vi "niccc-labview-xygraph.vi"() -> ()   [LabVIEW 2020]
uses:
  Controls/Frame Info (XY Graph).ctl
  Controls/Vertex.ctl
  Controls/State.ctl
panel:
  in  "FPS":u32=20
  in  "Slow Draw":bool
  out "Frame":i32
  out "XY Graph":cluster{"x":dbl[], "y":dbl[]}[](graph)
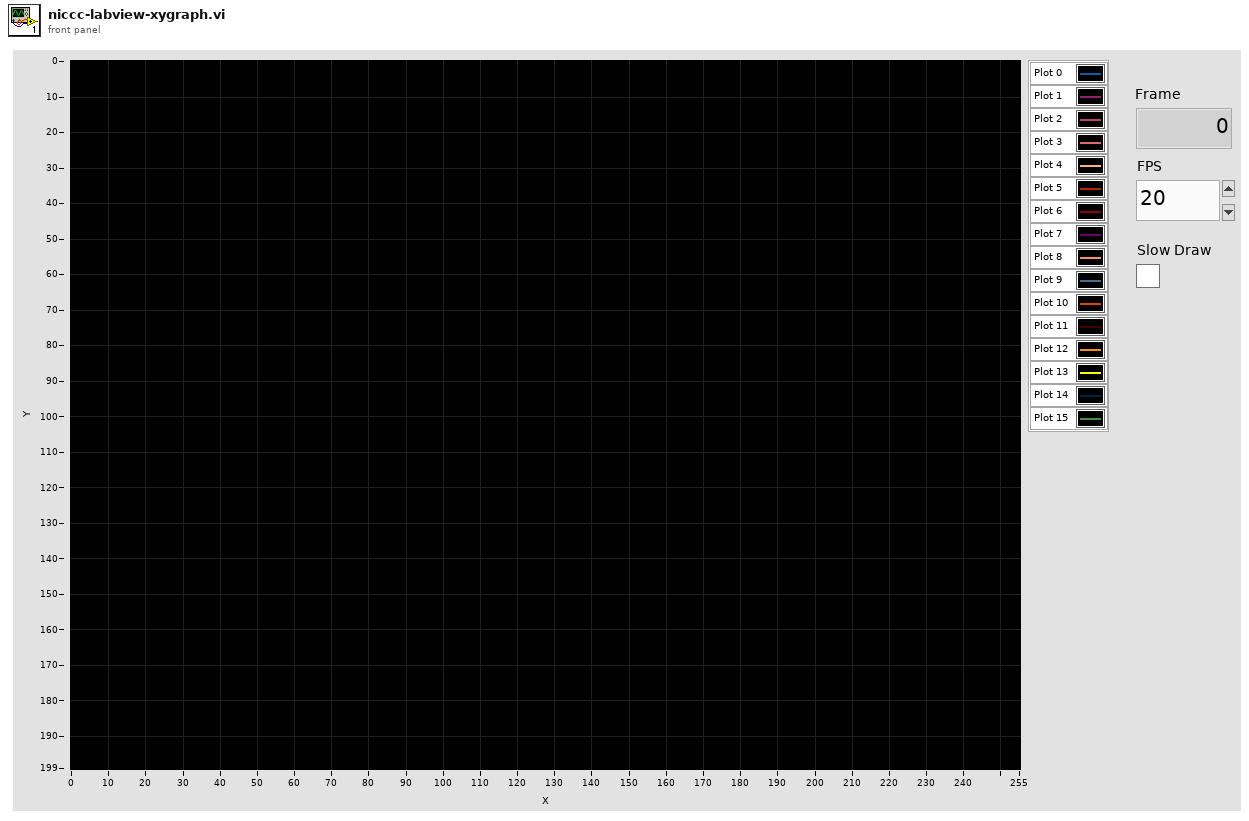
[diagram p1: front panel]
types:
  T1 = typedef "Frame Info (XY Graph).ctl" = cluster{"Clear Screen":bool, "Palette Data":bool, "Indexed":bool, "Indexed Verts":T2[], "Frame":i32, "Plots":cluster{"x":dbl[], "y":dbl[]}[]}
  T2 = typedef "Vertex.ctl" = cluster{"x":u8, "y":u8}
  T3 = typedef "State.ctl" = enum16{"Init", "Read Flags", "Clear Screen", "Update Palette", "Read Indexed", "Draw Polygons", "Skip 64kB", "Finish"}
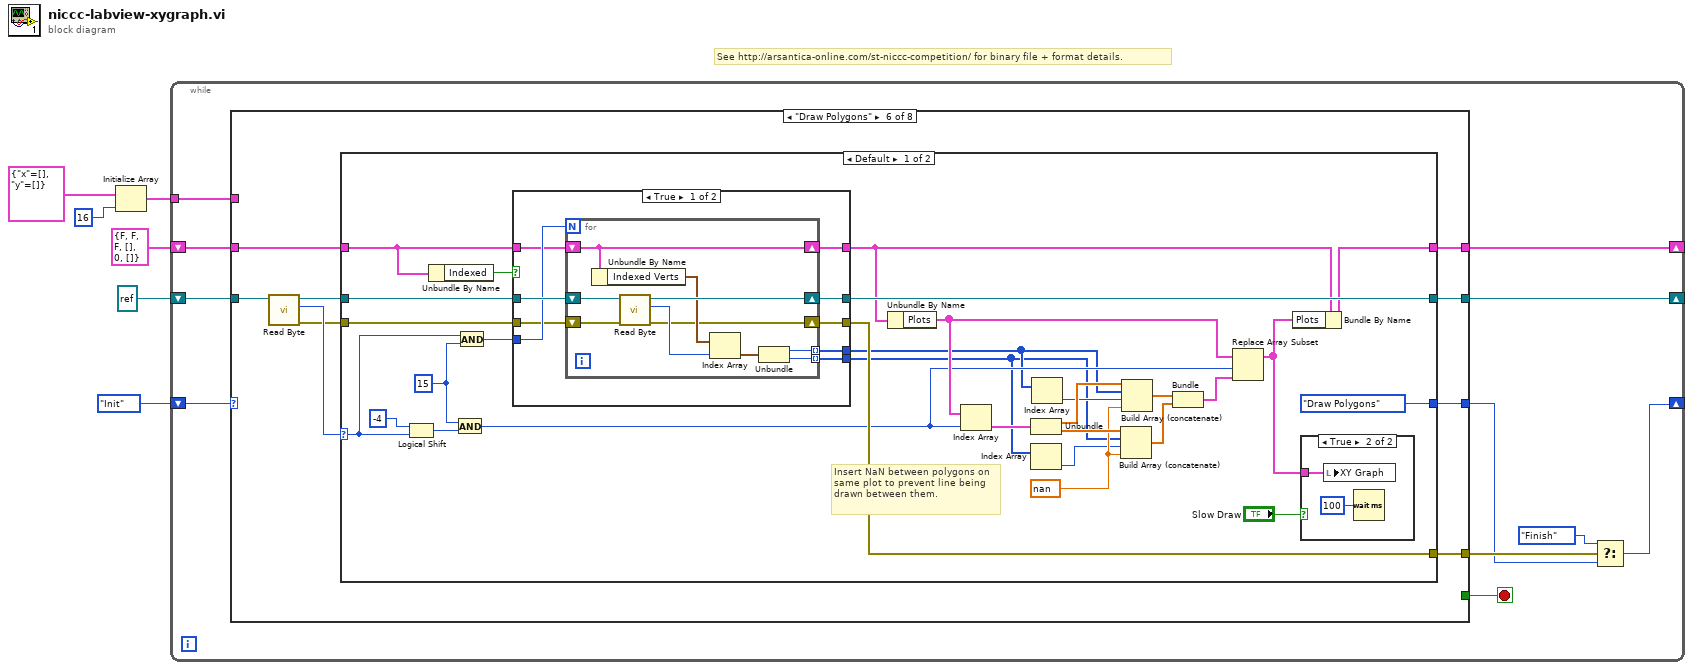
[diagram p0: block diagram]
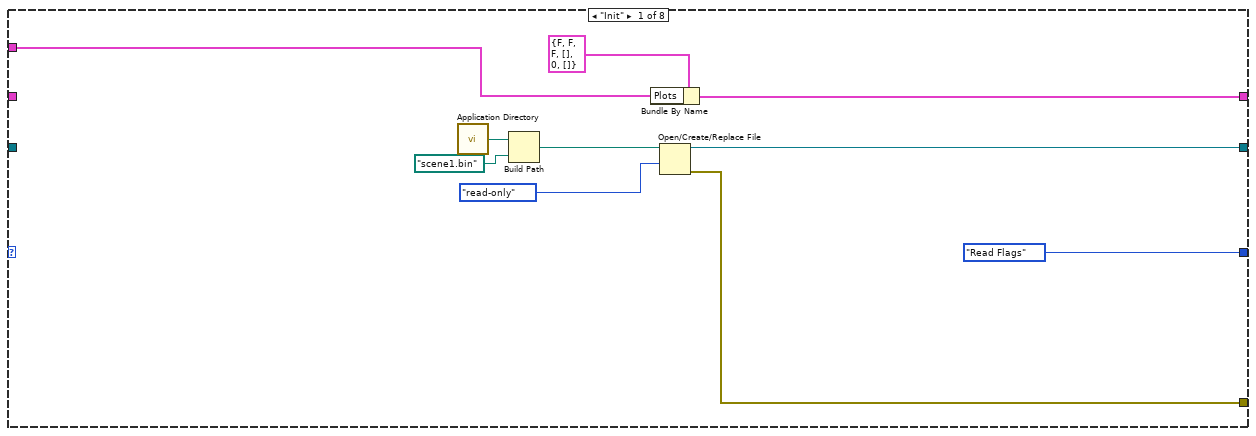
[diagram p2: hidden frame]
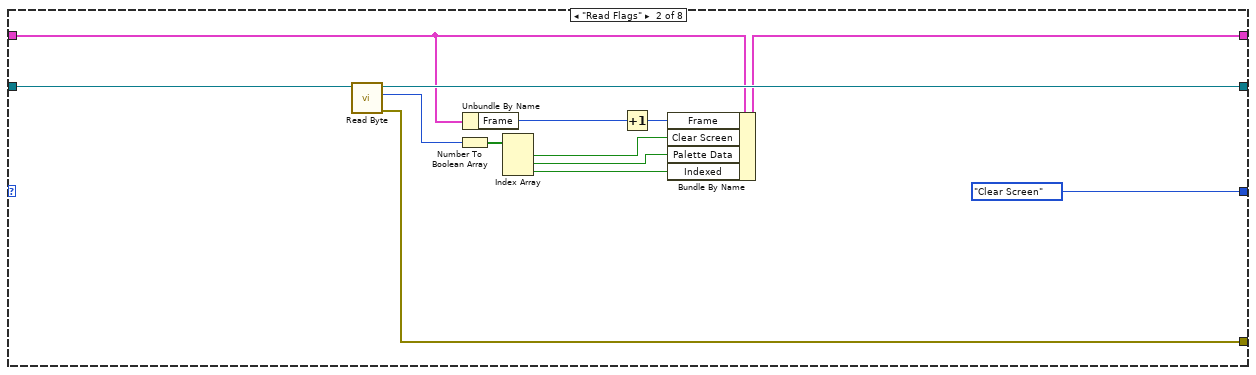
[diagram p3: hidden frame]
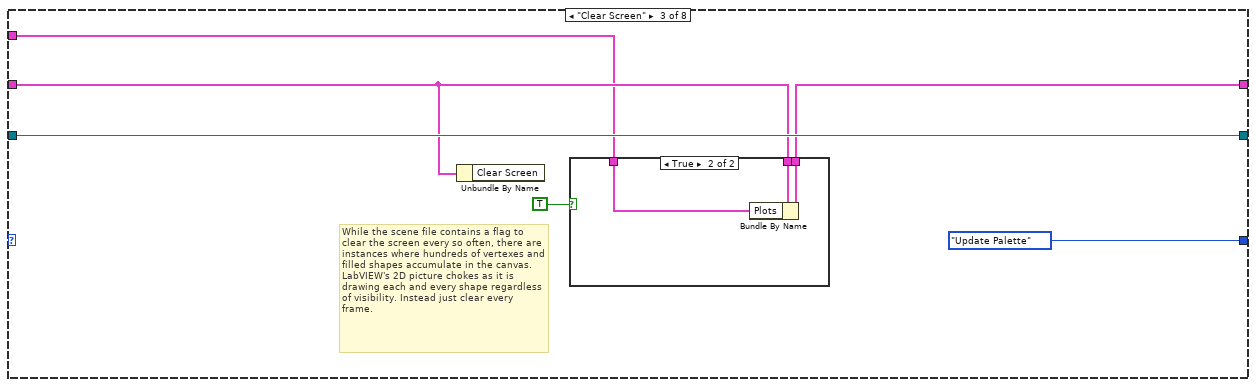
[diagram p4: hidden frame]
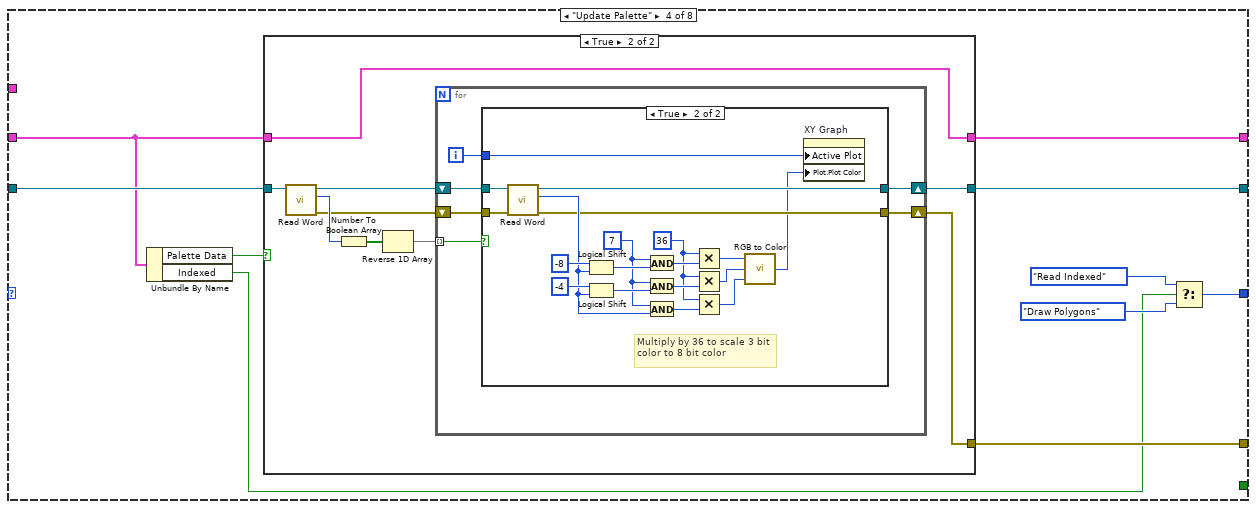
[diagram p6: hidden frame]
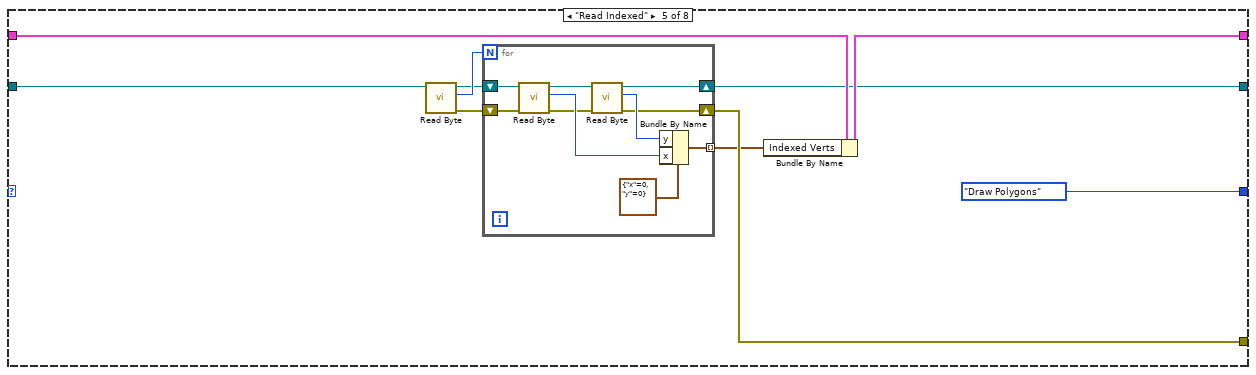
[diagram p9: hidden frame]
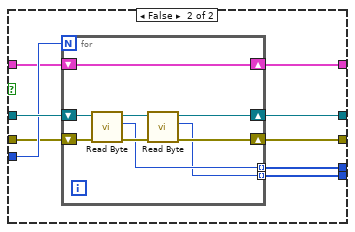
[diagram p11: hidden frame]
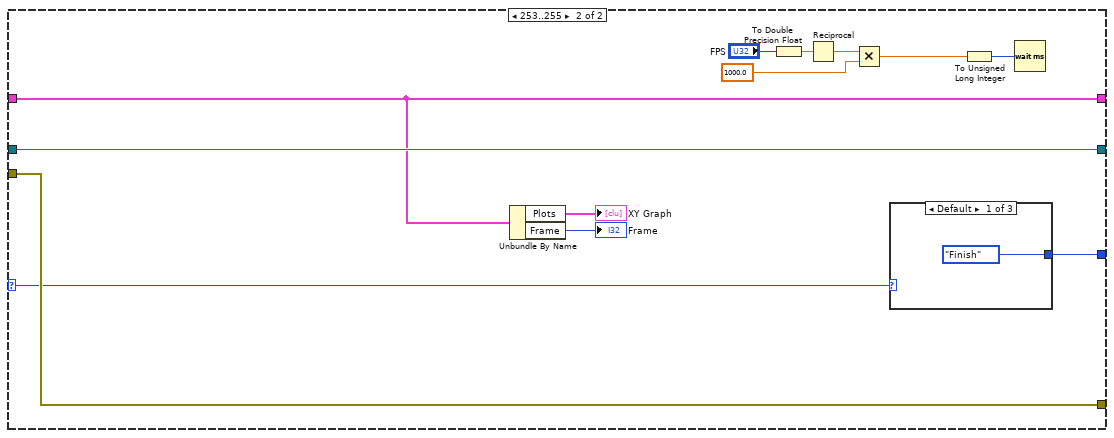
[diagram p12: hidden frame]
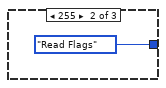
[diagram p13: hidden frame]
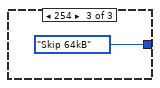
[diagram p14: hidden frame]
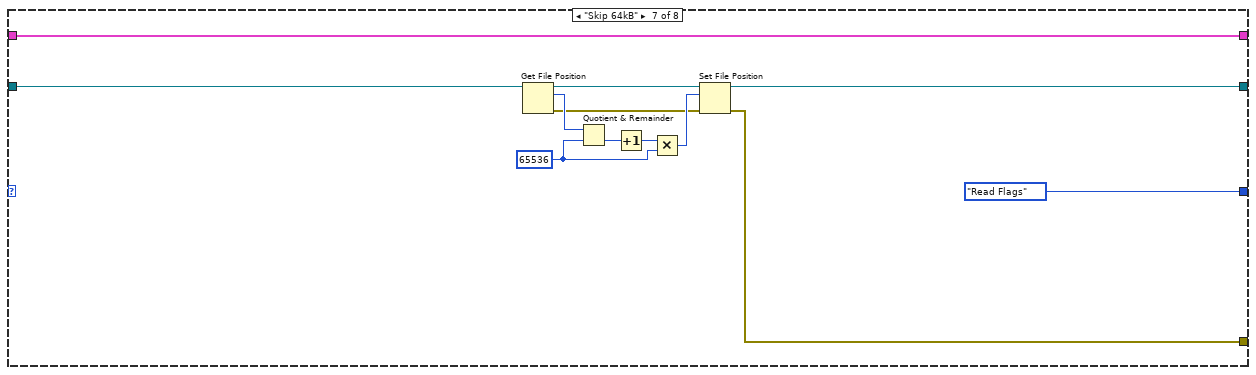
[diagram p15: hidden frame]
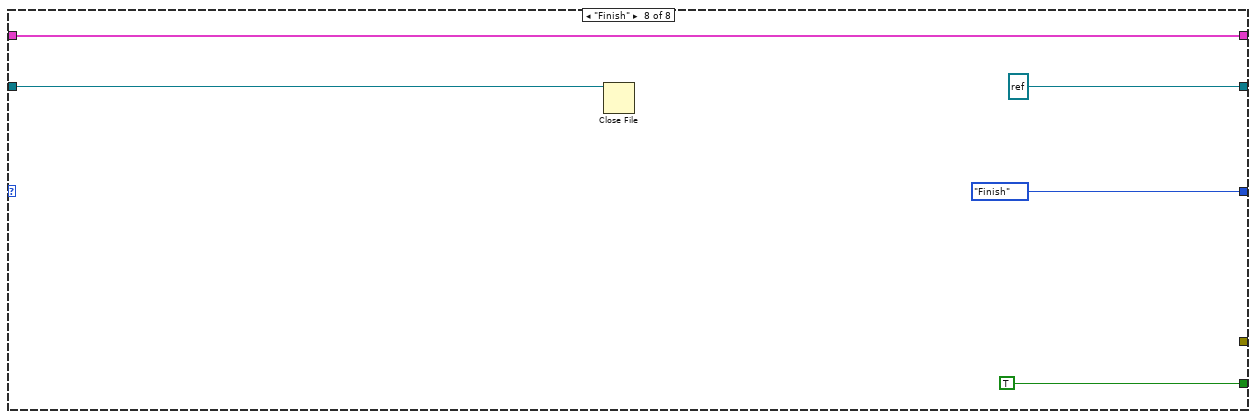
[diagram p16: hidden frame]
diagram:
  # "See http://arsantica-online.com/st-niccc-competition/ for binary file + format details."
  n1 = Initialize Array(cluster{"x":dbl[], "y":dbl[]} {"x"=[], "y"=[]} ("Plot"), 16) -> (w1:cluster{"x":dbl[], "y":dbl[]}[])
  n2 = while {
    shift-right: [w9] -> _
    shift-left: State."Init" -> [w17]
    shift-right: [w16] -> _
    shift-left: refnum<file> refnum ("refnum out") -> [w15]
    shift-right: [w13] -> _
    shift-left: T1 {"Clear Screen"=FALSE, "Palette Data"=FALSE, "Indexed"=FALSE, "Indexed Verts"=[], "Frame"=0, "Plots"=[]} -> [w14]
    tunnel: w1 -> [w7]
    stop <- w8 stop-if-true
    n3 = case shown="\"Draw Polygons\"" w17 {
      tunnel: [w23 w39 w46 w59 w103 w121 w218 refnum<file> refnum ("refnum out")] -> w16
      tunnel: w15 -> [_ w40 w46 w60 w108 w127 w219 w228]
      tunnel: w14 -> [_ w30 w44 w53 w104 w123 w223 w227]
      tunnel: [w22 w34 w45 w58 w105 w122 w223 w227] -> w13
      tunnel: [State."Read Flags" State."Clear Screen" State."Update Palette" w54 State."Draw Polygons" w125 State."Read Flags" State."Finish"] -> w10
      tunnel: [w21 w33 _ w57 w101 w119 w212 _] -> w11
      tunnel: [_ _ _ _ _ _ _ TRUE] -> w8
      tunnel: w7 -> [w18 _ w41 _ _ _ _ _]
      frame "Init" {
        n4 = call <vilib>:"Application Directory.vi"() -> ("Application Directory"=w27:path)
        n5 = Build Path(base path=w27, name or relative path=path "scene1.bin") -> (appended path=w25:path)
        n6 = Bundle By Name(cluster=T1 {"Clear Screen"=FALSE, "Palette Data"=FALSE, "Indexed"=FALSE, "Indexed Verts"=[], "Frame"=0, "Plots"=[]}, "Plots"=w18) -> (w22:T1)
        n7 = Open/Create/Replace File(file path (use dialog)=w25, access (0:read/write)=enum16{"read/write", "read-only", "write-only"}."read-only") -> (refnum out=w23:refnum<file>, error out=w21:errorcluster)  [unwired: 4 in, 1 out]
      }
      frame "Read Flags" {
        n8 = call "Read Byte.vi"("File Ref In"=w40) -> ("error out"=w33:errorcluster, "Word"=w38:u8, "File Ref Out"=w39:refnum<file>)  [unwired: 8 in]
        n9 = Number To Boolean Array(number=w38) -> (Boolean array=w37:bool[])
        n10 = Unbundle By Name(w30) -> ("Frame"=w29:i32)
        n11 = Index Array(array=w37) -> (element #1=w32:bool, element #2=w36:bool, element #3=w35:bool)  [unwired: 3 in]
        n12 = Increment(x=w29) -> (x+1=w28:i32)
        n13 = Bundle By Name(cluster=w30, "Frame"=w28, "Clear Screen"=w32, "Palette Data"=w36, "Indexed"=w35) -> (w34:T1)
      }
      frame "Clear Screen" {
        # "While the scene file contains a flag to clear the screen every so often, there are instances where hundreds of vertexes and filled shapes accumulate in the canvas. LabVIEW's 2D picture chokes as it is drawing each and every shape regardless of visibility. Instead just clear every frame."
        n14 = Unbundle By Name(w44) -> ()  [unwired: 1 out]
        n15 = case shown="True" TRUE {
          tunnel: w44 -> [w47 w50]
          tunnel: [w47 w49] -> w45
          tunnel: w41 -> [_ w48]
          frame False {
          }
          frame True {
            n16 = Bundle By Name(cluster=w50, "Plots"=w48) -> (w49:T1)
          }
        }
      }
      frame "Update Palette" {
        n17 = Unbundle By Name(w53) -> ("Palette Data"=w52:bool, "Indexed"=w51:bool)
        n18 = case shown="True" w52 {
          tunnel: w60 -> [w61 w71]
          tunnel: [w61 w67] -> w59
          tunnel: w53 -> [w62 w63]
          tunnel: [w62 w63] -> w58
          tunnel: [_ w64] -> w57
          frame False {
          }
          frame True {
            n19 = call "Read Word.vi"("File Ref In"=w71) -> ("error out"=w65:errorcluster, "Word"=w70:u16, "File Ref Out"=w68:refnum<file>)  [unwired: 8 in]
            n20 = Number To Boolean Array(number=w70) -> (Boolean array=w69:bool[])
            n21 = Reverse 1D Array(array=w69) -> (reversed array=w66:bool[])
            n22 = for {
              tunnel: w66 -> [w76] mode=indexing
              shift-right: [w75] -> w67
              shift-left: w68 -> [w77]
              shift-right: [w73] -> w64
              shift-left: w65 -> [w74]
              i -> [w72]
              n23 = case shown="True" w76 {
                tunnel: w77 -> [w79 w98]
                tunnel: [w79 w84] -> w75
                tunnel: w74 -> [w78 w83]
                tunnel: [w78 w82] -> w73
                tunnel: w72 -> [_ w81]
                frame False {
                }
                frame True {
                  w88 = u16 36 ("x")
                  w93 = u16 7 ("y")
                  # "Multiply by 36 to scale 3 bit color to 8 bit color"
                  n24 = call "Read Word.vi"("error in"=w83, "File Ref In"=w98) -> ("error out"=w82:errorcluster, "Word"=w92:u16, "File Ref Out"=w84:refnum<file>)  [unwired: 7 in]
                  n25 = Logical Shift(y=-8 ("x"), x=w92) -> (x << y=w95:u16)
                  n26 = Logical Shift(y=-4 ("x"), x=w92) -> (x << y=w94:u16)
                  n27 = And(x=w93, y=w95) -> (x .and. y?=w91:u16)
                  n28 = And(x=w93, y=w94) -> (x .and. y?=w89:u16)
                  n29 = And(x=w93, y=w92) -> (x .and. y?=w87:u16)
                  n30 = Multiply(x=w88, y=w91) -> (x*y=w90:u16)
                  n31 = Multiply(x=w88, y=w89) -> (x*y=w86:u16)
                  n32 = Multiply(x=w88, y=w87) -> (x*y=w85:u16)
                  n33 = call <vilib>:"RGB to Color.vi"("B"=w85, "G"=w86, "R"=w90) -> ("Color"=w80:u32)
                  n34 = property on="XY Graph" class="XYGraph (strict)"("Active Plot"=w81, "Plot.Plot Color"=w80) -> ()  [unwired: 2 in, 2 out]
                }
              }
            }
          }
        }
        n35 = Select(t=State."Read Indexed", s=w51, f=State."Draw Polygons") -> (s? t:f=w54:T3)
      }
      frame "Read Indexed" {
        n36 = call "Read Byte.vi"("File Ref In"=w108) -> ("error out"=w102:errorcluster, "Word"=w107:u8, "File Ref Out"=w106:refnum<file>)  [unwired: 8 in]
        n37 = for {
          N: w107 -> [_]
          shift-right: [w116] -> w103
          shift-left: w106 -> [w118]
          tunnel: [w115] -> w99 mode=indexing
          shift-right: [w109] -> w101
          shift-left: w102 -> [w111]
          n38 = call "Read Byte.vi"("error in"=w111, "File Ref In"=w118) -> ("error out"=w110:errorcluster, "Word"=w113:u8, "File Ref Out"=w117:refnum<file>)  [unwired: 7 in]
          n39 = call "Read Byte.vi"("error in"=w110, "File Ref In"=w117) -> ("error out"=w109:errorcluster, "Word"=w112:u8, "File Ref Out"=w116:refnum<file>)  [unwired: 7 in]
          n40 = Bundle By Name(cluster=T2 {"x"=0, "y"=0}, "y"=w112, "x"=w113) -> (w115:T2)
        }
        n41 = Bundle By Name(cluster=w104, "Indexed Verts"=w99) -> (w105:T1)
      }
      frame "Draw Polygons" {
        n42 = call "Read Byte.vi"("File Ref In"=w127) -> ("error out"=w120:errorcluster, "Word"=w126:u8, "File Ref Out"=w124:refnum<file>)  [unwired: 8 in]
        n43 = case shown="Default" w126 {
          selector: w126 -> [w153 w204]
          tunnel: [State."Draw Polygons" w208] -> w125
          tunnel: w124 -> [w150 w207]
          tunnel: w123 -> [w144 w206]
          tunnel: [w148 w206] -> w122
          tunnel: [w151 w207] -> w121
          tunnel: w120 -> [w146 w205]
          tunnel: [w145 w205] -> w119
          frame Default {
            w134 = nan
            w152 = u8 15 ("y")
            # "Insert NaN between polygons on same plot to prevent line being drawn between them."
            n44 = Logical Shift(y=i16 -4, x=w153) -> (x << y=w155:u8)
            n45 = Unbundle By Name(w144) -> ("Indexed"=w143:bool)
            n46 = And(x=w152, y=w155) -> (x .and. y?=w136:u8)
            n47 = And(x=w153, y=w152) -> (x .and. y?=w149:u8)
            n48 = case shown="True" w143 {
              tunnel: [w167 w186] -> w151
              tunnel: w150 -> [w166 w185]
              tunnel: w149 -> [w165 w184]
              tunnel: w144 -> [w164 w183]
              tunnel: [w160 w179] -> w130
              tunnel: [w163 w182] -> w147
              tunnel: w146 -> [w162 w181]
              tunnel: [w161 w180] -> w145
              tunnel: [w159 w178] -> w129
              frame True {
                n49 = for {
                  N: w165 -> [_]
                  shift-right: [w176] -> w167
                  shift-left: w166 -> [w177]
                  shift-right: [w173] -> w163
                  shift-left: w164 -> [w173]
                  tunnel: [w169] -> w160 mode=indexing
                  shift-right: [w171] -> w161
                  shift-left: w162 -> [w172]
                  tunnel: [w168] -> w159 mode=indexing
                  n50 = Unbundle By Name(w173) -> ("Indexed Verts"=w175:T2[])
                  n51 = call "Read Byte.vi"("error in"=w172, "File Ref In"=w177) -> ("error out"=w171:errorcluster, "Word"=w174:u8, "File Ref Out"=w176:refnum<file>)  [unwired: 7 in]
                  n52 = Index Array(array=w175, index=w174) -> (element=w170:T2)
                  n53 = Unbundle(w170) -> ("x"=w169:u8, "y"=w168:u8)
                }
              }
              frame False {
                n54 = for {
                  N: w184 -> [_]
                  shift-right: [w191] -> w186
                  shift-left: w185 -> [w195]
                  shift-right: [w194] -> w182
                  shift-left: w183 -> [w194]
                  shift-right: [w190] -> w180
                  shift-left: w181 -> [w193]
                  tunnel: [w188] -> w179 mode=indexing
                  tunnel: [w187] -> w178 mode=indexing
                  n55 = call "Read Byte.vi"("error in"=w193, "File Ref In"=w195) -> ("error out"=w189:errorcluster, "Word"=w188:u8, "File Ref Out"=w192:refnum<file>)  [unwired: 7 in]
                  n56 = call "Read Byte.vi"("error in"=w189, "File Ref In"=w192) -> ("error out"=w190:errorcluster, "Word"=w187:u8, "File Ref Out"=w191:refnum<file>)  [unwired: 7 in]
                }
              }
            }
            n57 = Unbundle By Name(w147) -> ("Plots"=w137:cluster{"x":dbl[], "y":dbl[]}[])
            n58 = Index Array(array=w137, index=w136) -> (element=w142:cluster{"x":dbl[], "y":dbl[]})
            n59 = Unbundle(w142) -> ("x"=w141:dbl[], "y"=w139:dbl[])
            n60 = Index Array(array=w129) -> (element=w128:u8)  [unwired: 1 in]
            n61 = Index Array(array=w130) -> (element=w133:u8)  [unwired: 1 in]
            n62 = Build Array (concatenate)(w139, w129, w128, w134) -> (w138:dbl[])
            n63 = Build Array (concatenate)(w141, w130, w133, w134) -> (w140:dbl[])
            n64 = Bundle(w140, w138) -> (w135:cluster{dbl[], dbl[]})  [unwired: 1 in]
            n65 = Replace Array Subset(array=w137, new element=w135, index=w136) -> (w132:cluster{"x":dbl[], "y":dbl[]}[])
            n66 = Bundle By Name(cluster=w147, "Plots"=w132) -> (w148:T1)
            n67 = case shown="True" "Slow Draw" {
              tunnel: w132 -> [_ w158]
              frame False {
              }
              frame True {
                n68 = local write "XY Graph"(w158) -> ()
                n69 = Wait (ms)(milliseconds to wait=u32 100) -> ()  [unwired: 1 out]
              }
            }
          }
          frame 253..255 {
            n70 = Unbundle By Name(w206) -> ("Plots"=→"XY Graph":cluster{"x":dbl[], "y":dbl[]}[], "Frame"=→"Frame":i32)
            n71 = To Double Precision Float(number="FPS") -> (double precision float=w202:dbl)
            n72 = Reciprocal(x=w202) -> (1/x=w198:dbl)
            n73 = Multiply(x=w198, y=1000.0) -> (x*y=w200:dbl)
            n74 = case shown="Default" w204 {
              tunnel: [State."Finish" State."Read Flags" State."Skip 64kB"] -> w208
              frame Default {
              }
              frame 255 {
              }
              frame 254 {
              }
            }
            n75 = To Unsigned Long Integer(number=w200) -> (unsigned 32bit integer=w197:u32)
            n76 = Wait (ms)(milliseconds to wait=w197) -> ()  [unwired: 1 out]
          }
        }
      }
      frame "Skip 64kB" {
        w215 = i64 65536 ("y")
        n77 = Get File Position(7:w219) -> (0:w213:errorcluster, 2:w221:i64, 3:w220:refnum<file>)  [unwired: 1 in]
        n78 = Quotient & Remainder(x=w221, y=w215) -> (floor(x/y)=w217:i64)  [unwired: 1 out]
        n79 = Increment(x=w217) -> (x+1=w216:i64)
        n80 = Multiply(x=w216, y=w215) -> (x*y=w214:i64)
        n81 = Set File Position(offset (in bytes) (0)=w214, refnum=w220, error in=w213) -> (refnum out=w218:refnum<file>, error out=w212:errorcluster)  [unwired: 1 in]
      }
      frame "Finish" {
        n82 = Close File(refnum=w228) -> ()  [unwired: 1 in, 2 out]
      }
    }
    n83 = Select(t=State."Finish", s=w11, f=w10) -> (s? t:f=w9:T3)
  }
